vi "OAT Get Slow Roll Vectors (N Channels).vi"(0 "scaled signals [EU]":waveform(dbl)[](array[waveform]), 1 "reference output mode":T1(ring), 2 "reset? (T)":bool=TRUE, 5 "speed profile":T2 {"speed [RPM]" format="%.2f"; "time [s]" format="%.2f"}, 7 "pulse/revolution (1)":i32=1, 9 "orders to compensate (1.0)":dbl[](array[numeric])=[1.0] format="%.2f", 11 "error in (no error)":errorcluster, 12 "bandwidth [order]":dbl format="%.2f") -> (4 "vector references":cdb[][](array[numeric]) format="%.2f", 15 "error out":errorcluster)   [LabVIEW 2017]
uses:
  <vilib>/addons/Sound and Vibration/Order Analysis/Tach Process/SubVIs/speed profile.ctl
  <vilib>/addons/Sound and Vibration/Order Analysis/Resample Order Tracking/OAT Order Magnitude and Phase (Even Angle Signal, N Channels).vi
  <vilib>/addons/Sound and Vibration/Order Analysis/Resample Order Tracking/OAT Convert to Even Angle Signal (N Channels).vi
  <vilib>/Analysis/NI_AALPro.lvlib
  <vilib>/addons/Sound and Vibration/Order Analysis/Resample Order Tracking/SoundVib_OrderTracking.lvlib
  <vilib>/addons/Sound and Vibration/Order Analysis/Tach Process/SoundVib_TachProcess.lvlib
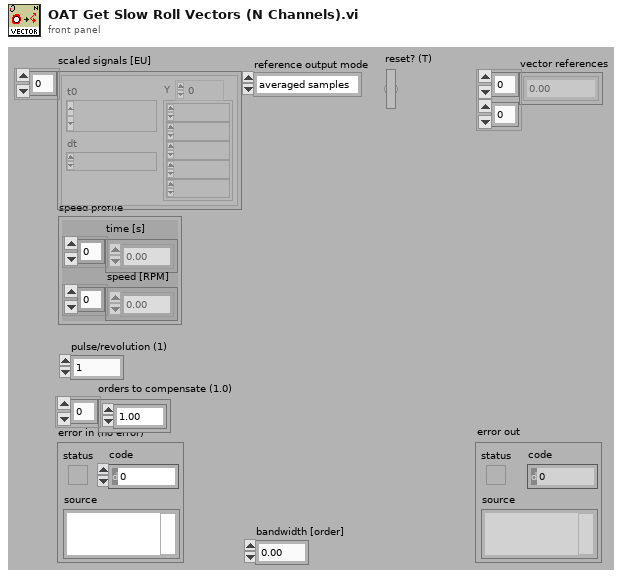
[diagram p1: front panel]
types:
  T1 = enum16{"averaged samples", "initial samples", "final samples"}
  T2 = typedef "SoundVib_TachProcess.lvlib/speed profile.ctl" = cluster{"time [s]":dbl[], "speed [RPM]":dbl[]}
  T3 = cluster{"dB on? (T)":bool, "unwrap phase? (T)":bool, "unit in degree? (T)":bool}
  T4 = typedef "svc_Resampled Channel Info.ctl" = cluster{"channel name":string, "description":string, " channel info":T5}
  T5 = typedef "svc_Channel Info.ctl" = cluster{"sensor sensitivity":dbl, "engineering units":T6, "dB reference":dbl, "custom label":string, "weighting filter":T7, "pregain":dbl}
  T6 = typedef "svc_Engineering Units Text Ring.ctl" = u16
  T7 = typedef "svc_Weighting Filter Text Ring.ctl" = u16
  T8 = typedef "OAT Position Info.ctl" = cluster{"positions [s]":dbl[], "samples/rev":dbl}
  T9 = cluster{"time/rev/rpm":dbl[], "magnitude":dbl[]}[][]
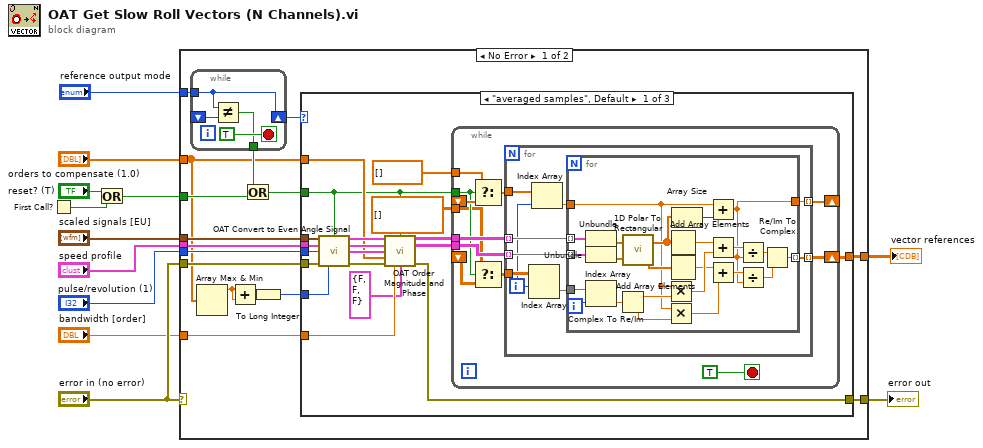
[diagram p0: block diagram]
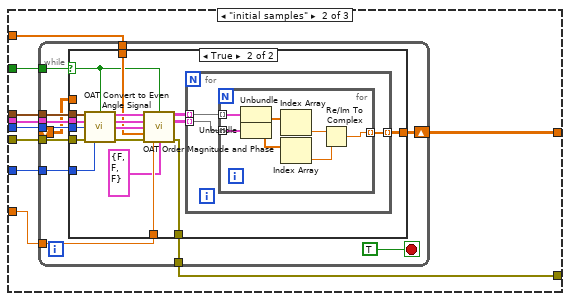
[diagram p2: hidden frame]
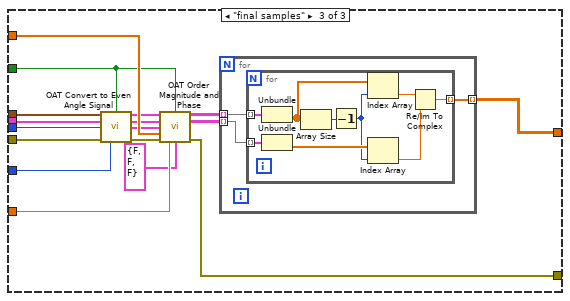
[diagram p4: hidden frame]
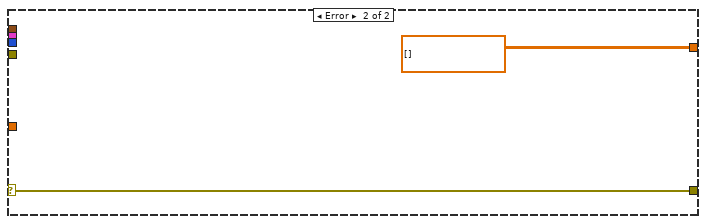
[diagram p5: hidden frame]
diagram:
  n1 = First Call?() -> (First Call?: T/F=w5:bool)
  n2 = Or(x="reset? (T)", y=w5) -> (x .or. y?=w4:bool)
  n3 = case shown="No Error" "error in (no error)" {
    selector: "error in (no error)" -> [_ w176]
    tunnel: "scaled signals [EU]" -> [w17 _]
    tunnel: "speed profile" -> [w28 _]
    tunnel: "pulse/revolution (1)" -> [w27 _]
    tunnel: "error in (no error)" -> [w26 _]
    tunnel: [w25 cdb[][] []] -> w9
    tunnel: [w24 w176] -> w8
    tunnel: w4 -> [w20 _]
    tunnel: "bandwidth [order]" -> [w23 _]
    tunnel: "orders to compensate (1.0)" -> [w14 _]
    tunnel: "reference output mode" -> [w22 _]
    frame No Error {
      n4 = while {
        shift-right: [w32] -> w21
        shift-left: _ -> [w31]
        tunnel: w22 -> [w32]
        tunnel: [w29] -> w19
        stop <- TRUE stop-if-true
        n5 = Not Equal?(x=w32, y=w31) -> (x != y?=w29:bool)
      }
      n6 = Array Max & Min(array=w14) -> (max value=w16:dbl)  [unwired: 3 out]
      n7 = Add(x=w16, y=w16) -> (x+y=w15:dbl)
      n8 = Or(x=w19, y=w20) -> (x .or. y?=w18:bool)
      n9 = To Long Integer(number=w15) -> (32bit integer=w13:i32)
      n10 = case shown="\"averaged samples\", Default" w21 {
        tunnel: w17 -> [w51 w105 w163]
        tunnel: w28 -> [w50 w104 w162]
        tunnel: w27 -> [w49 w103 w161]
        tunnel: w26 -> [w48 w102 w160]
        tunnel: [w38 w101 w159] -> w25
        tunnel: [w43 w100 w158] -> w24
        tunnel: w23 -> [w42 w99 w157]
        tunnel: w14 -> [w41 w98 w156]
        tunnel: w18 -> [w35 w97 w149]
        tunnel: w13 -> [w34 w96 w148]
        frame "averaged samples", Default {
          n11 = call-poly <vilib>:"OAT Convert to Even Angle Signal.vi"("scaled signals [EU]"=w51, "reset? (F)"=w35, "speed profile"=w50, "pulse/revolution (1)"=w49, "error in (no error)"=w48, "max order (auto)"=w34) -> ("even-angle signals"=w47:cluster{"r0":dbl, "dr":dbl, "Y":dbl[]}[], "even-angle channel info"=w46:T4[], "even-angle position info"=w45:T8, "error out"=w44:errorcluster)  [unwired: 5 in, 1 out]
          n12 = call-poly <vilib>:"OAT Order Magnitude and Phase.vi"("even-angle signals"=w47, "reset? (F)"=w35, "even-angle channel info"=w46, "even-angle position info"=w45, "orders to compute (1.0)"=w41, "error in (no error)"=w44, "bandwidth [order]"=w42, "view"=T3 {"dB on? (T)"=FALSE, "unwrap phase? (T)"=FALSE, "unit in degree? (T)"=FALSE}) -> ("magnitudes [RMS]"=w40:T9, "phases [phase lag]"=w39:cluster{"time/rev/rpm":dbl[], "phase":dbl[]}[][], "error out"=w43:errorcluster)  [unwired: 2 in, 3 out]
          n13 = while {
            tunnel: w40 -> [w63]
            tunnel: w39 -> [w62]
            shift-right: [w59] -> _
            shift-left: _ -> [w58]
            shift-right: [w60] -> w38
            shift-left: _ -> [w56]
            tunnel: w35 -> [w54]
            tunnel: dbl[] [] -> [w55]
            tunnel: cdb[][] [] -> [w52]
            stop <- TRUE stop-if-true
            n14 = Select(t=w55, s=w54, f=w58) -> (s? t:f=w57:dbl[])
            n15 = Select(t=w52, s=w54, f=w56) -> (s? t:f=w53:cdb[][])
            n16 = for {
              tunnel: w63 -> [w72] mode=indexing
              tunnel: w62 -> [w71] mode=indexing
              tunnel: [w70] -> w60 mode=indexing
              tunnel: [w69] -> w59 mode=indexing
              tunnel: w57 -> [w66]
              tunnel: w53 -> [w68]
              i -> [w65]
              n17 = Index Array(array=w68, index (row)=w65) -> (element=w67:cdb[])  [unwired: 1 in]
              n18 = Index Array(array=w66, index=w65) -> (element=w64:dbl)
              n19 = for {
                tunnel: w72 -> [w95] mode=indexing
                tunnel: w71 -> [w94] mode=indexing
                tunnel: [w92] -> w70 mode=indexing
                tunnel: [w79] -> w69
                tunnel: w67 -> [w76]
                tunnel: w64 -> [w73]
                i -> [w74]
                n20 = Unbundle(w95) -> ("magnitude"=w93:dbl[])  [unwired: 1 out]
                n21 = Unbundle(w94) -> ("phase"=w91:dbl[])  [unwired: 1 out]
                n22 = Index Array(array=w76, index=w74) -> (element=w75:cdb)
                n23 = Complex To Re/Im(x + iy=w75) -> (x=w89:dbl, y=w88:dbl)
                n24 = call <vilib>:"1D Polar To Rectangular.vi"("Magnitude"=w93, "Phase"=w91) -> ("X"=w87:dbl[], "Y"=w86:dbl[])  [unwired: 1 out]
                n25 = Multiply(x=w73, y=w89) -> (x*y=w84:dbl)
                n26 = Multiply(x=w73, y=w88) -> (x*y=w82:dbl)
                n27 = Add Array Elements(numeric array=w87) -> (sum=w85:dbl)
                n28 = Add Array Elements(numeric array=w86) -> (sum=w83:dbl)
                n29 = Array Size(array=w87) -> (size(s)=w90:i32)
                n30 = Add(x=w73, y=w90) -> (x+y=w79:dbl)
                n31 = Add(x=w85, y=w84) -> (x+y=w81:dbl)
                n32 = Add(x=w83, y=w82) -> (x+y=w80:dbl)
                n33 = Divide(x=w81, y=w79) -> (x/y=w78:dbl)
                n34 = Divide(x=w80, y=w79) -> (x/y=w77:dbl)
                n35 = Re/Im To Complex(1:w77, 2:w78) -> (0:w92:cdb)
              }
            }
          }
        }
        frame "initial samples" {
          n36 = while {
            tunnel: w105 -> [w117]
            tunnel: w104 -> [w116]
            tunnel: w103 -> [w115]
            tunnel: w102 -> [w114]
            tunnel: [w112] -> w100
            tunnel: w99 -> [w111]
            tunnel: w98 -> [w110]
            tunnel: w97 -> [w109]
            shift-right: [w113] -> w101
            shift-left: _ -> [w107]
            tunnel: w96 -> [w106]
            stop <- TRUE stop-if-true
            n37 = case shown="True" w109 {
              selector: w109 -> [_ w122]
              tunnel: w117 -> [_ w136]
              tunnel: w116 -> [_ w135]
              tunnel: w115 -> [_ w134]
              tunnel: w114 -> [w118 w133]
              tunnel: [w119 w126] -> w113
              tunnel: [w118 w125] -> w112
              tunnel: w111 -> [_ w124]
              tunnel: w110 -> [_ w123]
              tunnel: w107 -> [w119 _]
              tunnel: w106 -> [_ w121]
              frame False {
              }
              frame True {
                n38 = call-poly <vilib>:"OAT Convert to Even Angle Signal.vi"("scaled signals [EU]"=w136, "reset? (F)"=w122, "speed profile"=w135, "pulse/revolution (1)"=w134, "error in (no error)"=w133, "max order (auto)"=w121) -> ("even-angle signals"=w132:cluster{"r0":dbl, "dr":dbl, "Y":dbl[]}[], "even-angle channel info"=w131:T4[], "even-angle position info"=w130:T8, "error out"=w129:errorcluster)  [unwired: 5 in, 1 out]
                n39 = call-poly <vilib>:"OAT Order Magnitude and Phase.vi"("even-angle signals"=w132, "reset? (F)"=w122, "even-angle channel info"=w131, "even-angle position info"=w130, "orders to compute (1.0)"=w123, "error in (no error)"=w129, "bandwidth [order]"=w124, "view"=T3 {"dB on? (T)"=FALSE, "unwrap phase? (T)"=FALSE, "unit in degree? (T)"=FALSE}) -> ("magnitudes [RMS]"=w128:T9, "phases [phase lag]"=w127:cluster{"time/rev/rpm":dbl[], "phase":dbl[]}[][], "error out"=w125:errorcluster)  [unwired: 2 in, 3 out]
                n40 = for {
                  tunnel: w128 -> [w139] mode=indexing
                  tunnel: w127 -> [w138] mode=indexing
                  tunnel: [w137] -> w126 mode=indexing
                  n41 = for {
                    tunnel: w139 -> [w146] mode=indexing
                    tunnel: w138 -> [w145] mode=indexing
                    tunnel: [w144] -> w137 mode=indexing
                    n42 = Unbundle(w146) -> ("magnitude"=w143:dbl[])  [unwired: 1 out]
                    n43 = Unbundle(w145) -> ("phase"=w142:dbl[])  [unwired: 1 out]
                    n44 = Index Array(array=w143) -> (element=w141:dbl)  [unwired: 1 in]
                    n45 = Index Array(array=w142) -> (element=w140:dbl)  [unwired: 1 in]
                    n46 = Re/Im To Complex(1:w140, 2:w141) -> (0:w144:cdb)
                  }
                }
              }
            }
          }
        }
        frame "final samples" {
          n47 = call-poly <vilib>:"OAT Convert to Even Angle Signal.vi"("scaled signals [EU]"=w163, "reset? (F)"=w149, "speed profile"=w162, "pulse/revolution (1)"=w161, "error in (no error)"=w160, "max order (auto)"=w148) -> ("even-angle signals"=w155:cluster{"r0":dbl, "dr":dbl, "Y":dbl[]}[], "even-angle channel info"=w154:T4[], "even-angle position info"=w153:T8, "error out"=w152:errorcluster)  [unwired: 5 in, 1 out]
          n48 = call-poly <vilib>:"OAT Order Magnitude and Phase.vi"("even-angle signals"=w155, "reset? (F)"=w149, "even-angle channel info"=w154, "even-angle position info"=w153, "orders to compute (1.0)"=w156, "error in (no error)"=w152, "bandwidth [order]"=w157, "view"=T3 {"dB on? (T)"=FALSE, "unwrap phase? (T)"=FALSE, "unit in degree? (T)"=FALSE}) -> ("magnitudes [RMS]"=w151:T9, "phases [phase lag]"=w150:cluster{"time/rev/rpm":dbl[], "phase":dbl[]}[][], "error out"=w158:errorcluster)  [unwired: 2 in, 3 out]
          n49 = for {
            tunnel: w151 -> [w166] mode=indexing
            tunnel: w150 -> [w165] mode=indexing
            tunnel: [w164] -> w159 mode=indexing
            n50 = for {
              tunnel: w166 -> [w175] mode=indexing
              tunnel: w165 -> [w174] mode=indexing
              tunnel: [w173] -> w164 mode=indexing
              n51 = Unbundle(w175) -> ("magnitude"=w168:dbl[])  [unwired: 1 out]
              n52 = Unbundle(w174) -> ("phase"=w172:dbl[])  [unwired: 1 out]
              n53 = Array Size(array=w168) -> (size(s)=w169:i32)
              n54 = Decrement(x=w169) -> (x-1=w167:i32)
              n55 = Index Array(array=w168, index=w167) -> (element=w171:dbl)
              n56 = Index Array(array=w172, index=w167) -> (element=w170:dbl)
              n57 = Re/Im To Complex(1:w170, 2:w171) -> (0:w173:cdb)
            }
          }
        }
      }
    }
    frame Error {
    }
  }
  "error out" <- w8
  "vector references" <- w9
